vi "CAPS_acquisition.vi"() -> ()   [LabVIEW 2017]
uses:
  <vilib>/Utility/error.llb/DialogType.ctl
  <vilib>/DAQmx/write.llb/DAQmx Write (Digital Wfm 1Chan NSamp).vi
  <vilib>/DAQmx/write.llb/DAQmx Write (Analog 1D Wfm NChan NSamp).vi
  <vilib>/DAQmx/create/channels.llb/DAQmx Create Channel (AO-Voltage-Basic).vi
  <vilib>/DAQmx/configure/timing.llb/DAQmx Timing (Sample Clock).vi
  <vilib>/DAQmx/miscellaneous.llb/DAQmx Fill In Error Info.vi
  <vilib>/DAQmx/create/channels.llb/DAQmx Create Channel (DO-Digital Output).vi
  <vilib>/Waveform/DWDTOps.llb/DWDT Analog to Digital.vi
  <vilib>/DAQmx/configure/trigger.llb/DAQmx Start Trigger (Digital Edge).vi
  <vilib>/Waveform/DWDTOps.llb/DWDT Uncompress Digital.vi
  <resource>/objmgr/daqmx.rc
  <vilib>/measure/NI_MABase.lvlib
panel:
  in  "Cam Delay (s)":dbl=0.5
  in  "CR":dbl=15.0
  in  "Vgalvo sine":T1={"frequency"=50.0, "amplitude"=0.068, "offset"=0.0, "phase"=118.0}
  in  "Vetl sine":T1={"frequency"=50.0, "amplitude"=0.8, "offset"=2.0, "phase"=0.0}
  in  "Camera start trigger phase":dbl=63.0
  in  "DO Retrigger Physical Source":tag="/PXI1Slot3_2/PFI3"
  in  "DO Sample Clock Source":tag="OnboardClock"
  in  "DMD DO Physical Channel":tag="PXI1Slot3_2/port0/line0"
  in  "Logging Mode":i32(ring)=10231 items=["Off"=10231, "Log and Read"=15842]
  out "error out":errorcluster
  in  "Folder Name":string="nucGFP_3dpf_1st_1"
  in  "Root Path":path=path "D:/Data/Zebrafish/05262025_1"
  in  "Total Frames":i32=1100
  out "Frames Recorded":i32
  in  "Exposure Time(s)":dbl=0.00199
  in  "Sub Region":T2={"Horizontal Offset"=1020, "Vertical Offset"=820, "Horizontal Size"=580, "Vertical Size"=404}
  in  "AO Number of Samples":i32=400000
  in  "AO Sample Clock Source":tag="OnboardClock"
  in  "AO Physical Channels":tag="PXI1Slot3_2/ao29, PXI1Slot3_2/ao31,  PXI1Slot3_2/ao3"
  # "Layser analogue out: \ngreen ao0: 10\ngreen ao0 GND: 11\nblue ao1: 44\nblue ao1 GND: 11"
  # "galvo analogue out: \nao29: 66\nao29 GND: 33"
  # "ETL analogue out:\nao31: 34\nao31 GND: 68"
  # "Camera start analogue out: \nao3: 12\nao3 GND: 46"
  # "DMD retriggerable digital out: \ndo P0.0: 2\ndo P0.0 GND: 36\n\nDigital trigger source: \ndi PFI 3: 6\ndi PFI 2 GND: 39"
  # "DMD digital in: \ndi P0.1: 3\ndi P0.1 GND: 36"
  # "1072\n820\n596\n404"
  # "5Hz\n0.07268   0.7\n0.29948   2\n173.4       0"
  # "50Hz\n0.0718   0.8\n0.298   2\n115.56     0"
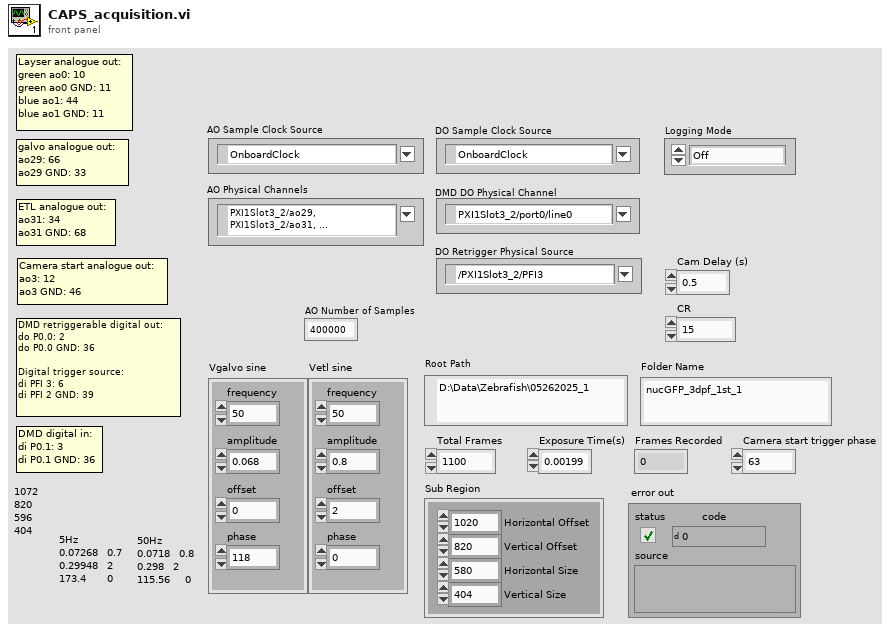
[diagram p1: front panel]
types:
  T1 = cluster{"frequency":dbl, "amplitude":dbl, "offset":dbl, "phase":dbl}
  T2 = cluster{"Horizontal Offset":i32, "Vertical Offset":i32, "Horizontal Size":i32, "Vertical Size":i32}
  T3 = typedef "DialogType.ctl" = u16
  T4 = enum16{"open", "replace", "create", "open or create", "replace or create", "replace or create with confirmation"}
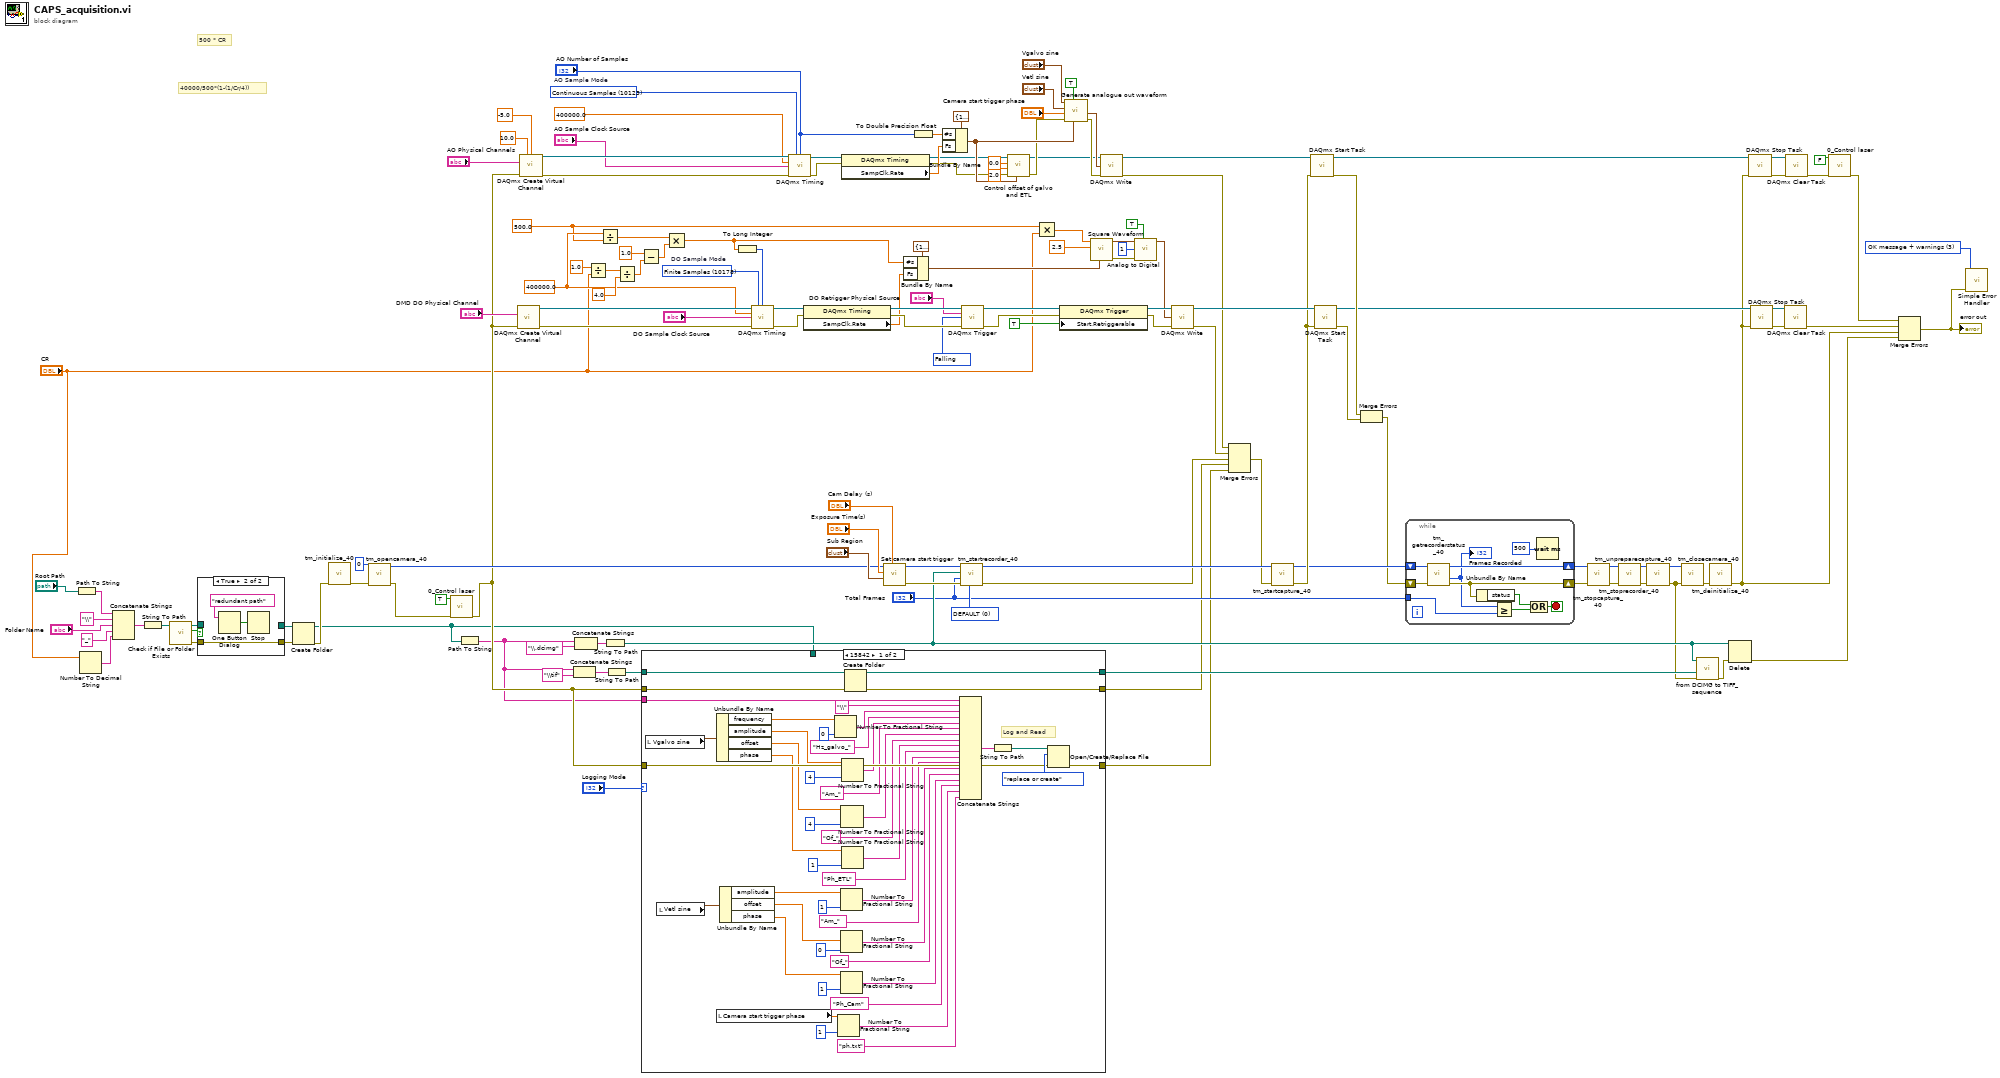
[diagram p0: block diagram]
diagram:
  w17 = 400000.0 ("DO Sample Rate")
  w92 = 10171 items=["Rising"=10280, "Falling"=10171] ("Edge")
  w15 = 500.0
  w53 = T3 3 items=["no dialog", "OK message", "continue or stop message", "OK message + warnings", "continue/stop + warnings"] ("type of dialog (OK msg:1)")
  w100 = 10178 items=["Finite Samples"=10178, "Continuous Samples"=10123, "Hardware Timed Single Point"=12522]  # DO Sample Mode
  w120 = 0 items=["DEFAULT", "NO BUFFERING"] ("Buffering Mode")
  w137 = 10123 items=["Finite Samples"=10178, "Continuous Samples"=10123, "Hardware Timed Single Point"=12522]  # AO Sample Mode
  # "40000/500*(1-(1/Cr/4))"
  # "500 * CR"
  n1 = Path To String(path="Root Path") -> (string=w83:string)
  n2 = Number To Decimal String(number="CR") -> (decimal integer string=w1:string)  [unwired: 1 in]
  n3 = Concatenate Strings(w83, "\\", "Folder Name", "_", w1) -> (w80:string)
  n4 = String To Path(string=w80) -> (path=w74:path)
  n5 = call <vilib>:"Check if File or Folder Exists.vi"("path"=w74) -> ("error out"=w70:errorcluster, "file or folder exists?"=w75:bool, "dup path"=w76:path)  [unwired: 8 in]
  n6 = case shown="True" w75 {
    tunnel: w76 -> [w142 _]
    tunnel: [w142 _] -> w73
    tunnel: w70 -> [w141 w143]
    tunnel: [w141 w143] -> w69
    frame False {
    }
    frame True {
      n7 = One Button Dialog(message="redundant path") -> (true=w144:bool)  [unwired: 1 in]
      n8 = Stop(stop? (T)=w144) -> ()
    }
  }
  n9 = Create Folder(path (use dialog)=w73, error in=w69) -> (created path=w36:path, error out=w42:errorcluster)  [unwired: 1 in, 1 out]
  n10 = call <userlib>:"tm_initialize_40.vi"("error in (no error)"=w42) -> ("error out"=w128:errorcluster)  [unwired: 7 in, 3 out]
  n11 = call <userlib>:"tm_opencamera_40.vi"("error in (no error)"=w128, "Camera Index"=u32 0) -> ("error out"=w13:errorcluster, "Handle out"=w41:u32)  [unwired: 7 in, 1 out]
  n12 = call "0_Control laser.vi"("error in (no error)"=w13, "Laser On/Off"=TRUE) -> ("error out"=w38:errorcluster)  [unwired: 9 in]
  n13 = Path To String(path=w36) -> (string=w26:string)
  n14 = call-poly <vilib>:"DAQmx Create Virtual Channel.vi"("lines"="DMD DO Physical Channel", "error in"=w38) -> ("task out"=w102:refnum<k21>, "error out"=w101:errorcluster)  [unwired: 12 in]
  n15 = call-poly <vilib>:"DAQmx Create Virtual Channel.vi"("maximum value"=10.0 ("AO Max Voltage"), "minimum value"=-5.0 ("AO Min Voltage"), "physical channels"="AO Physical Channels", "error in"=w38) -> ("task out"=w135:refnum<k21>, "error out"=w136:errorcluster)  [unwired: 10 in]
  n16 = Concatenate Strings(w26, "\\tif") -> (w72:string)
  n17 = Concatenate Strings(w26, "\\.dcimg") -> (w77:string)
  n18 = Divide(x=1.0, y="CR") -> (x/y=w22:dbl)
  n19 = Divide(x=w17, y=w15) -> (x/y=w25:dbl)
  n20 = String To Path(string=w77) -> (path=w71:path)
  n21 = String To Path(string=w72) -> (path=w39:path)
  n22 = Divide(x=w22, y=4.0) -> (x/y=w20:dbl)
  n23 = Subtract(x=1.0, y=w20) -> (x-y=w19:dbl)
  n24 = case shown="15842" "Logging Mode" {
    tunnel: w38 -> [w189 w193]
    tunnel: [w188 w193] -> w30
    tunnel: w39 -> [w187 _]
    tunnel: w38 -> [w186 w192]
    tunnel: [w185 w191] -> w37
    tunnel: [w184 w192] -> w31
    tunnel: w36 -> [_ w191]
    tunnel: w26 -> [w146 _]
    frame 15842 {
      # "Log and Read"
      n25 = local read "Vgalvo sine"() -> (w173:T1)
      n26 = local read "Vetl sine"() -> (w178:T1)
      n27 = local read "Camera start trigger phase"() -> (w182:dbl)
      n28 = Unbundle By Name(w173) -> ("frequency"=w174:dbl, "amplitude"=w175:dbl, "offset"=w176:dbl, "phase"=w177:dbl)
      n29 = Unbundle By Name(w178) -> ("amplitude"=w179:dbl, "offset"=w180:dbl, "phase"=w181:dbl)
      n30 = Number To Fractional String(number=w174, precision (6)=0) -> (F-format string=w166:string)  [unwired: 2 in]
      n31 = Number To Fractional String(number=w182, precision (6)=1) -> (F-format string=w183:string)  [unwired: 2 in]
      n32 = Number To Fractional String(number=w179, precision (6)=1) -> (F-format string=w169:string)  [unwired: 2 in]
      n33 = Number To Fractional String(number=w180, precision (6)=0) -> (F-format string=w170:string)  [unwired: 2 in]
      n34 = Number To Fractional String(number=w181, precision (6)=1) -> (F-format string=w171:string)  [unwired: 2 in]
      n35 = Number To Fractional String(number=w176, precision (6)=4) -> (F-format string=w168:string)  [unwired: 2 in]
      n36 = Number To Fractional String(number=w175, precision (6)=4) -> (F-format string=w167:string)  [unwired: 2 in]
      n37 = Number To Fractional String(number=w177, precision (6)=1) -> (F-format string=w148:string)  [unwired: 2 in]
      n38 = Create Folder(path (use dialog)=w187, error in=w186) -> (created path=w185:path, error out=w184:errorcluster)  [unwired: 1 in, 1 out]
      n39 = Concatenate Strings(w146, "\\", w166, "Hz_galvo_", w167, "Am_", w168, "Of_", w148, "Ph_ETL", w169, "Am_", w170, "Of_", w171, "Ph_Cam", w183, "ph.txt") -> (w172:string)
      n40 = String To Path(string=w172) -> (path=w147:path)
      n41 = Open/Create/Replace File(file path (use dialog)=w147, error in=w189, operation (0:open)=T4."replace or create") -> (error out=w188:errorcluster)  [unwired: 3 in, 2 out]
    }
    frame 10231, Default {
      # "Off"
    }
  }
  n42 = Multiply(x=w25, y=w19) -> (x*y=w16:dbl)
  n43 = To Long Integer(number=w16) -> (32bit integer=w18:i32)
  n44 = call-poly <vilib>:"DAQmx Timing.vi"("task/channels in"=w102, "sample mode"=w100, "samples per channel"=w18, "rate"=w17, "source"="DO Sample Clock Source", "error in"=w101) -> ("task out"=w99:refnum<k21>, "error out"=w98:errorcluster)  [unwired: 8 in]
  n45 = call-poly <vilib>:"DAQmx Timing.vi"("task/channels in"=w135, "sample mode"=w137, "samples per channel"="AO Number of Samples", "rate"=400000.0 ("AO Sample Rate"), "source"="AO Sample Clock Source", "error in"=w136) -> ("task out"=w113:refnum<k21>, "error out"=w112:errorcluster)  [unwired: 8 in]
  n46 = property class="DAQmx Timing"(reference=w99, error in=w98) -> (reference out=w97:refnum<k21>, error out=w96:errorcluster, "SampClk.Rate"=w68:dbl)
  n47 = property class="DAQmx Timing"(reference=w113, error in=w112) -> (reference out=w8:refnum<k21>, error out=w11:errorcluster, "SampClk.Rate"=w111:dbl)
  n48 = call "Set camera start trigger.vi"("Cam Delay"="Cam Delay (s)", "Sub Region"="Sub Region", "Exposure Time(s)"="Exposure Time(s)", "Handle in"=w41) -> ("error out"=w119:errorcluster, "Handle out"=w122:u32)  [unwired: 6 in]
  n49 = Bundle By Name(cluster=cluster{"Fs":dbl, "#s":dbl} {"Fs"=1000.0, "#s"=1000.0} ("sampling info"), "#s"=w16, "Fs"=w68) -> (w85:cluster{"Fs":dbl, "#s":dbl})
  n50 = To Double Precision Float(number="AO Number of Samples") -> (double precision float=w129:dbl)
  n51 = Bundle By Name(cluster=cluster{"Fs":dbl, "#s":dbl} {"Fs"=1000.0, "#s"=1000.0} ("sampling info"), "#s"=w129, "Fs"=w111) -> (w12:cluster{"Fs":dbl, "#s":dbl})
  n52 = call <userlib>:"tm_startrecorder_40.vi"("Buffering Mode"=w120, "error in (no error)"=w119, "frames"="Total Frames", "File"=w71, "Handle in"=w122) -> ("error out"=w32:errorcluster, "Handle out"=w121:u32)  [unwired: 5 in]
  n53 = call-poly <vilib>:"DAQmx Trigger.vi"("task/channels in"=w97, "source"="DO Retrigger Physical Source", "edge"=w92, "error in"=w96) -> ("task out"=w90:refnum<k21>, "error out"=w88:errorcluster)  [unwired: 10 in]
  n54 = call "Control offset of galvo and ETL.vi"("sampling info"=w12, "error in (no error)"=w11, "ETL offset"=2.0, "Galvo offset"=0.0, "task/channels in"=w8) -> ("error out"=w10:errorcluster, "task out"=w7:refnum<k21>)  [unwired: 5 in]
  n55 = Multiply(x=w15, y="CR") -> (x*y=w14:dbl)
  n56 = property class="DAQmx Trigger"(reference=w90, error in=w88, "Start.Retriggerable"=TRUE) -> (reference out=w89:refnum<k21>, error out=w67:errorcluster)
  n57 = call "Generate analogue out waveform.vi"("sampling info"=w12, "Reset signal"=TRUE, "error in (no error)"=w10, "Camera start trigger phase"="Camera start trigger phase", "Vetl sine"="Vetl sine", "Vgalvo sine"="Vgalvo sine") -> ("error out"=w9:errorcluster, "Waveform Graph"=w57:waveform(dbl)[])  [unwired: 4 in]
  n58 = call <vilib>:"Square Waveform.vi"("sampling info"=w85, "amplitude"=2.5, "frequency"=w14) -> ("error out"=w108:errorcluster, "signal out"=w86:waveform(dbl))  [unwired: 7 in]
  n59 = call-poly <vilib>:"DAQmx Write.vi"("task/channels in"=w7, "data"=w57, "error in"=w9) -> ("task out"=w138:refnum<k21>, "error out"=w59:errorcluster)  [unwired: 10 in, 1 out]
  n60 = call-poly <vilib>:"Analog to Digital.vi"("compress digital (T)"=TRUE, "error in (no error)"=w108, "resolution (16 bit)"=1, "analog waveform"=w86) -> ("digital waveform"=w47:digitalwaveform)  [unwired: 4 in, 3 out]
  n61 = call-poly <vilib>:"DAQmx Write.vi"("task/channels in"=w89, "data"=w47, "error in"=w67) -> ("task out"=w95:refnum<k21>, "error out"=w60:errorcluster)  [unwired: 10 in, 1 out]
  n62 = Merge Errors(w59, w60, w32, w31, w30) -> (w58:errorcluster)
  n63 = call <userlib>:"tm_startcapture_40.vi"("error in (no error)"=w58, "Handle in"=w121) -> ("error out"=w66:errorcluster, "Handle out"=w51:u32)  [unwired: 8 in]
  n64 = call <vilib>:"DAQmx Start Task.vi"("task/channels in"=w138, "error in"=w66) -> ("task out"=w116:refnum<k21>, "error out"=w65:errorcluster)  [unwired: 12 in]
  n65 = call <vilib>:"DAQmx Start Task.vi"("task/channels in"=w95, "error in"=w66) -> ("task out"=w63:refnum<k21>, "error out"=w64:errorcluster)  [unwired: 12 in]
  n66 = Merge Errors(w65, w64) -> (w50:errorcluster)
  n67 = while {
    tunnel: "Total Frames" -> [w201]
    shift-right: [w203] -> w48
    shift-left: w51 -> [w202]
    shift-right: [w200] -> w33
    shift-left: w50 -> [w198]
    stop <- w195 stop-if-true
    n68 = call <userlib>:"tm_getrecorderstatus_40.vi"("error in (no error)"=w198, "Handle"=w202) -> ("error out"=w200:errorcluster, "Count"=w199:i32, "Handle"=w203:u32)  [unwired: 6 in, 1 out]
    "Frames Recorded" <- w199
    n69 = Unbundle By Name(w200) -> ("status"=w197:bool)
    n70 = Greater Or Equal?(x=w199, y=w201) -> (x >= y?=w196:bool)
    n71 = Compound Arithmetic op=OR(w197, w196) -> (w195:bool)
    n72 = Wait (ms)(milliseconds to wait=u32 500) -> ()  [unwired: 1 out]
  }
  n73 = call <userlib>:"tm_stopcapture_40.vi"("error in (no error)"=w33, "Handle in"=w48) -> ("error out"=w61:errorcluster, "Handle out"=w123:u32)  [unwired: 8 in]
  n74 = call <userlib>:"tm_stoprecorder_40.vi"("error in (no error)"=w61, "Handle in"=w123) -> ("error out"=w52:errorcluster, "Handle out"=w124:u32)  [unwired: 8 in]
  n75 = call <userlib>:"tm_unpreparecapture_40.vi"("error in (no error)"=w52, "Handle in"=w124) -> ("error out"=w35:errorcluster, "Handle out"=w114:u32)  [unwired: 8 in]
  n76 = call <userlib>:"tm_closecamera_40.vi"("error in (no error)"=w35, "Handle in"=w114) -> ("error out"=w115:errorcluster)  [unwired: 9 in]
  n77 = call "from DCIMG to TIFF_sequence.vi"("error in (no error)"=w35, "Where to Store"=w37, "DCIMG Path"=w71) -> ("Error Out"=w110:errorcluster)  [unwired: 7 in, 1 out]
  n78 = call <userlib>:"tm_deinitialize_40.vi"("error in (no error)"=w115) -> ("error out"=w34:errorcluster)  [unwired: 10 in]
  n79 = Delete(path (use dialog)=w71, error in=w110) -> (error out=w29:errorcluster)  [unwired: 3 in, 2 out]
  n80 = call <vilib>:"DAQmx Stop Task.vi"("task/channels in"=w116, "error in"=w34) -> ("task out"=w140:refnum<k21>, "error out"=w139:errorcluster)  [unwired: 12 in]
  n81 = call <vilib>:"DAQmx Stop Task.vi"("task/channels in"=w63, "error in"=w34) -> ("task out"=w94:refnum<k21>, "error out"=w93:errorcluster)  [unwired: 12 in]
  n82 = call <vilib>:"DAQmx Clear Task.vi"("task in"=w94, "error in"=w93) -> ("error out"=w62:errorcluster)  [unwired: 13 in]
  n83 = call <vilib>:"DAQmx Clear Task.vi"("task in"=w140, "error in"=w139) -> ("error out"=w28:errorcluster)  [unwired: 13 in]
  n84 = call "0_Control laser.vi"("error in (no error)"=w28, "Laser On/Off"=FALSE) -> ("error out"=w27:errorcluster)  [unwired: 9 in]
  n85 = Merge Errors(w27, w62, w34, w29) -> (w43:errorcluster)
  "error out" <- w43
  n86 = call <vilib>:"Simple Error Handler.vi"("type of dialog (OK msg:1)"=w53, "error in (no error)"=w43) -> ()  [unwired: 3 in, 5 out]
